vi "connectNodes.vi"(0 "reference":refnum<class "Graph.lvclass">, 1 "egde":refnum<class "AbstractEdge.lvclass">, 2 "start":refnum<class "AbstractNode.lvclass">, 3 "end":refnum<class "AbstractNode.lvclass">, 5 "error in (no error)":errorcluster) -> (14 "reference out":refnum<class "Graph.lvclass">, 15 "connected":bool, 19 "error out":errorcluster)   [LabVIEW 2012, in "Graph.lvclass"]
doc: "/**\n Adds an edge to this graph. This method should\n only be called by a decoder when reading a data file.\n @param e the edge to add\n @param start the start node of the edge\n @param end the end node of the edge\n */\n public void connect(Edge e, Node start, Node end)\n {\n e.connect(start, end);\n edges.add(e);\n }"
uses:
  <resource>/Framework/Providers/Open_GDS/UML/Graph_class/Graph.lvclass
  <resource>/Framework/Providers/Open_GDS/UML/AbstractEdge_class/AbstractEdge.lvclass
  <resource>/Framework/Providers/Open_GDS/UML/AbstractNode_class/AbstractNode.lvclass
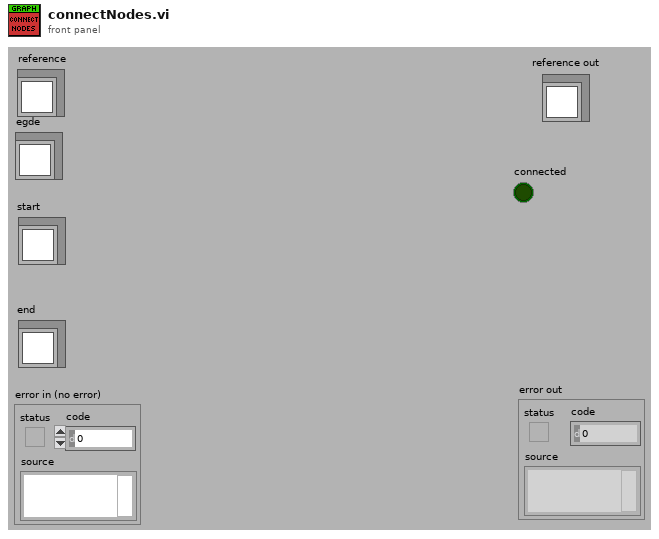
[diagram p1: front panel]
types:
  T1 = typedef "Graph.lvclass/ObjectAttributes.ctl" = cluster{"nodes":refnum<class "AbstractNode.lvclass">[], "edges":refnum<class "AbstractEdge.lvclass">[], "nodesToBeRemoved":refnum<class "AbstractNode.lvclass">[], "edgesToBeRemoved":refnum<class "AbstractEdge.lvclass">[], "needsLayout":bool, "LayoutNodes":refnum<class "AbstractNode.lvclass">[]}
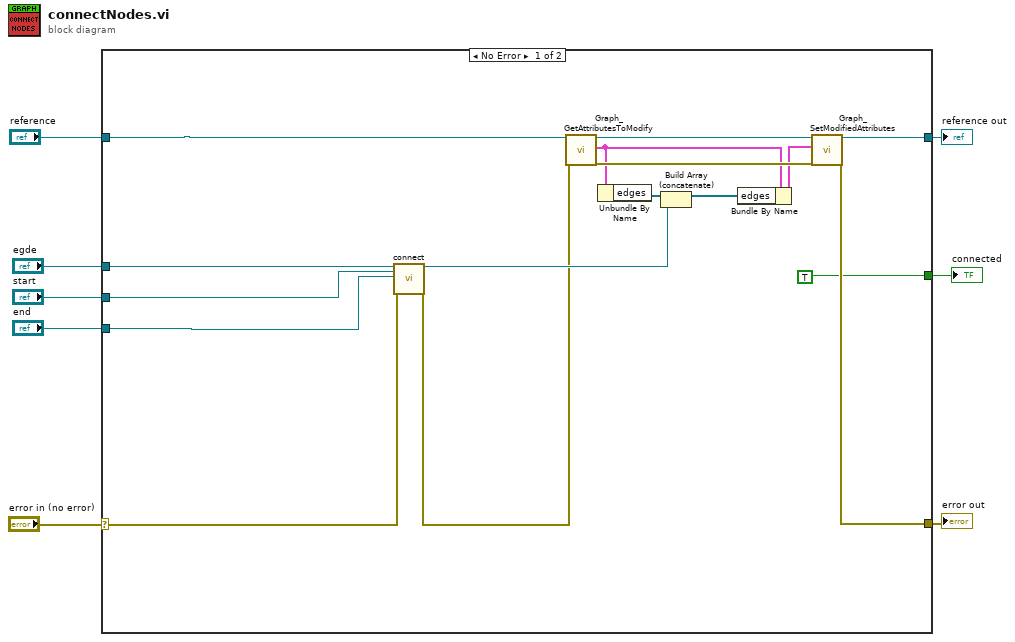
[diagram p0: block diagram]
diagram:
  n1 = case shown="No Error" "error in (no error)" {
    selector: "error in (no error)" -> [w21 w25]
    tunnel: "reference" -> [w24 w26]
    tunnel: [w23 w25] -> w7
    tunnel: [w22 w26] -> w6
    tunnel: "egde" -> [w20 _]
    tunnel: "start" -> [w19 _]
    tunnel: "end" -> [w18 _]
    tunnel: [TRUE ("needsLayout") _] -> w1
    frame No Error {
      n2 = call-dynamic "connect.vi"("reference"=w20, "startNode"=w19, "endNode"=w18, "error in (no error)"=w21) -> ("reference out"=w10:refnum<class "AbstractEdge.lvclass">, "error out"=w9:errorcluster)  [unwired: 14 out]
      n3 = call <resource>:"Graph_GetAttributesToModify.vi"("reference in"=w24, "error in (no error)"=w9) -> ("reference out"=w16:refnum<class "Graph.lvclass">, "Attributes"=w13:T1, "error out"=w15:errorcluster)  [unwired: 1 in, 14 out]
      n4 = Unbundle By Name(w13) -> ("edges"=w12:refnum<class "AbstractEdge.lvclass">[])
      n5 = Build Array (concatenate)(w12, w10) -> (w11:refnum<class "AbstractEdge.lvclass">[])
      n6 = Bundle By Name(cluster=w13, "edges"=w11) -> (w14:T1)
      n7 = call <resource>:"Graph_SetModifiedAttributes.vi"("reference in"=w16, "Attributes"=w14, "error in (no error)"=w15) -> ("reference out"=w22:refnum<class "Graph.lvclass">, "error out"=w23:errorcluster)  [unwired: 3 in, 12 out]
    }
    frame Error {
    }
  }
  "reference out" <- w6
  "error out" <- w7
  "connected" <- w1
